vi "FPGA Time Management.vi"   [LabVIEW 2020]
uses:
  <vilib>/Platform/TimedLoop/XDataNode/timing_clust.ctl
  <vilib>/Platform/TimedLoop/XDataNode/nitl_modes.ctl
  <vilib>/Platform/TimedLoop/XDataNode/wakeup.ctl
  <vilib>/rvi/Emulation/niFpgaGetClockAttributes.vi
  <vilib>/rvi/Emulation/niFpgaSctlEmulationGetInTimedLoop.vi
  <vilib>/rvi/Emulation/niFpgaEmulationReportErrorSimple.vi
  <vilib>/rvi/eio/common/nirviEmuTemplateMethod_errors.vi
  <vilib>/rvi/eio/common/nirviEmuTemplatePropertyGet_noerrors.vi
  Front Panel Globals.vi
  <vilib>/rvi/Emulation/niFpgaProcessEmulError.vi
  <vilib>/rvi/Emulation/niFpgaCriticalErrorInLSC.vi
  <vilib>/eio/EIOMethodNode/EIOMethodNode.xnode
  <vilib>/eio/EIOPropertyNode/EIOPropertyNode.xnode
  <vilib>/LabVIEW Targets/FPGA/cRIO/shared/nicrio_ModuleControls/nicrio_cRIO-9467_Latitude.ctl
  <vilib>/LabVIEW Targets/FPGA/cRIO/shared/nicrio_ModuleControls/nicrio_cRIO-9467_Longitude.ctl
  <vilib>/LabVIEW Targets/FPGA/cRIO/shared/nicrio_ModuleControls/nicrio_cRIO-9467_Altitude.ctl
  <vilib>/platform/TimedLoop/XDataNode/XDataNode.xnode
  FPGA Timekeeper 1.1b0/FPGA Timekeeper.lvlib
  <vilib>/rvi/eio/common/nirviEmuTemplatePropertyGet_errors.vi
  <vilib>/rvi/eio/common/nirviEmuTemplatePropertySet_errors.vi
  <vilib>/rvi/eio/common/nirviEmuTemplatePropertySet_noerrors.vi
  <vilib>/Platform/TimedLoop/XDataNode/XDNodeRunTimeDep.lvlib
types:
  T1 = typedef "XDNodeRunTimeDep.lvlib/timing_clust.ctl" = cluster{"Expected End [f-1]":u64, "Actual End [f-1]":u64, "Finished Late? [f-1]":bool, "Expected End [i-1]":u64, "Actual End [i-1]":u64, "Finished Late? [i-1]":bool, "Expected Start [i]":u64, "Actual Start [i]":u64, "Expected Start [f]":u64, "Actual Start [f]":u64, "Source Name":string, "Structure Name":string, "Period":i64, "Deadline":i64, "Offset":i64, "Start":i64, "Priority":i32, "Timeout":i32, "Mode":T2, "Wakeup Reason":T3, "Error":errorcluster, "Source Type":string, "Secondary Source Type":string, "Global End Time":u64, "Global Start Time":u64, "Frame Duration":u64, "Iteration Duration":u64, "Assigned CPU":i32, "I/O Scan Engine Mode":u32}
  T2 = typedef "XDNodeRunTimeDep.lvlib/nitl_modes.ctl" = enum32{"No Change", "Process missed periods, maintain original phase", "Discard missed periods, maintain original phase", "Process missed periods, ignore original phase", "Discard missed periods, ignore original phase"}
  T3 = typedef "XDNodeRunTimeDep.lvlib/wakeup.ctl" = enum32{"Normal", "Aborted", "Asynchronous wakeup", "Timing source error", "Timed loop error", "Timeout"}
  T4 = enum8{"Initializing", "Normal", "Unable to get fix"}
  T5 = enum8{"Unknown", "Normal", "Absent", "Overcurrent"}
  T6 = typedef "nicrio_cRIO-9467_Latitude.ctl" = fxp<+/-,28,8>
  T7 = typedef "nicrio_cRIO-9467_Longitude.ctl" = fxp<+/-,29,9>
  T8 = typedef "nicrio_cRIO-9467_Altitude.ctl" = fxp<+/-,24,17>
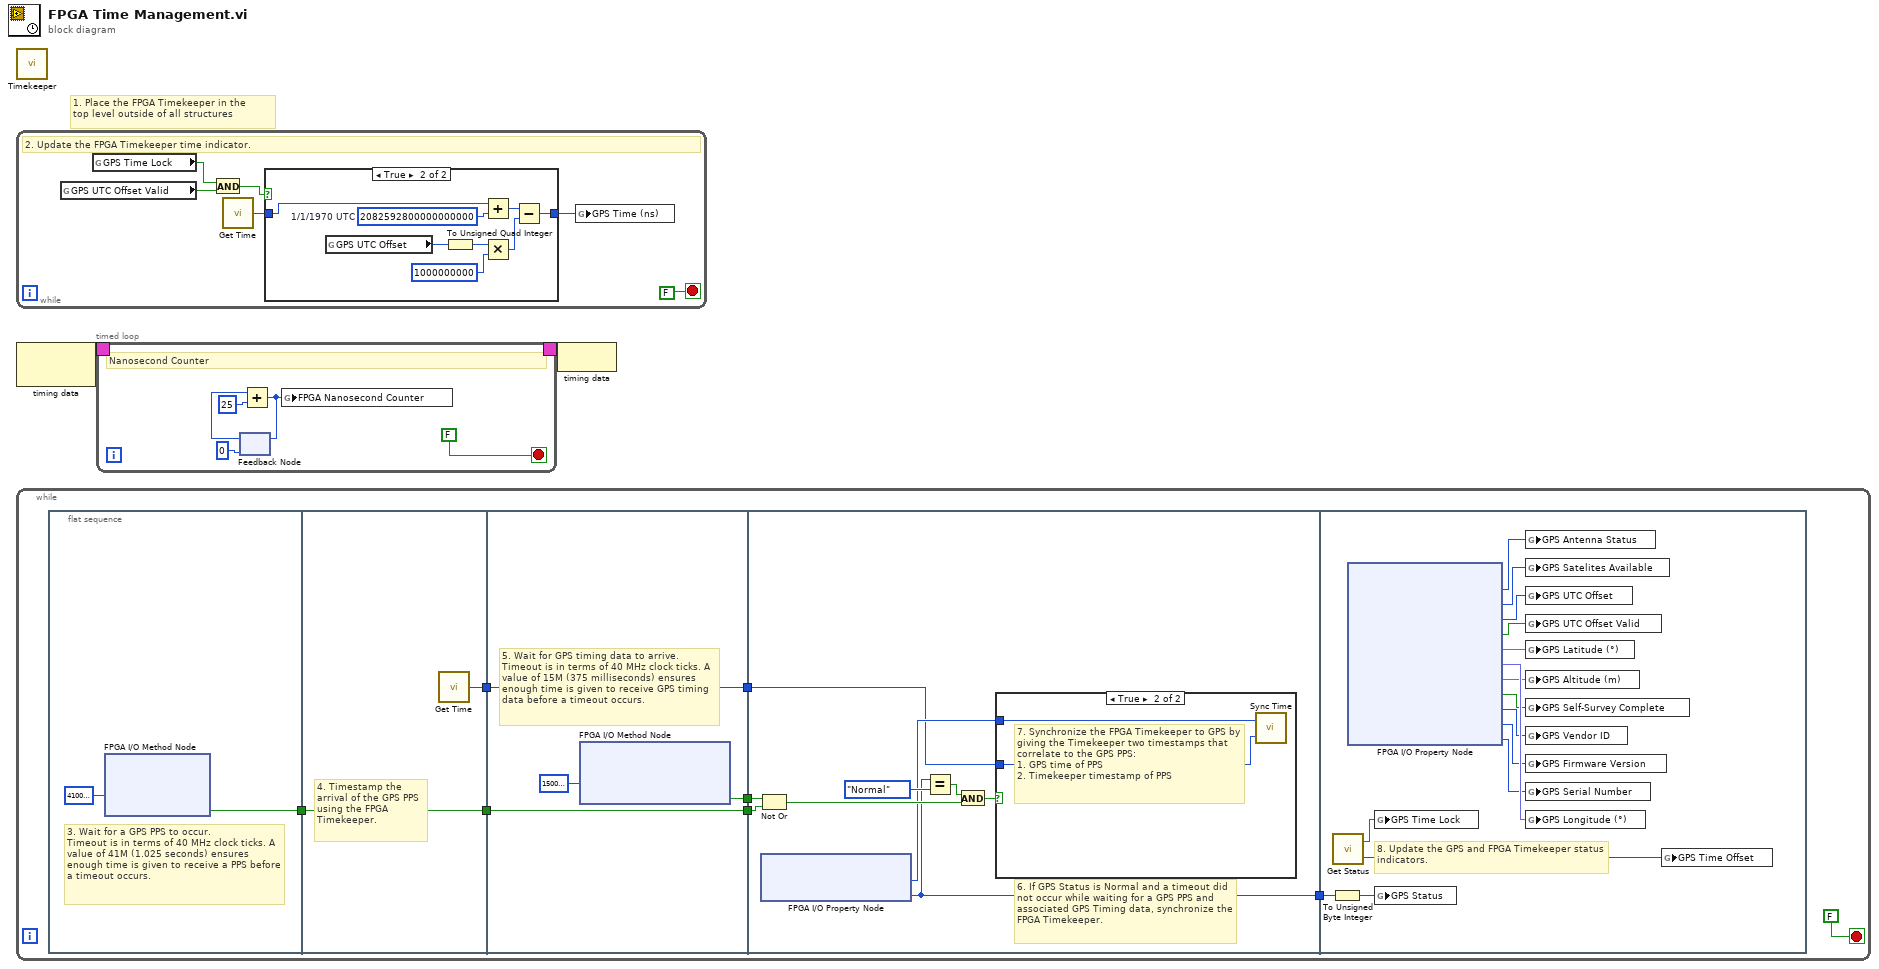
[diagram p0: block diagram]
diagram:
  # "1. Place the FPGA Timekeeper in the\ntop level outside of all structures"
  n1 = call "Timekeeper.vi"() -> ()  [unwired: 12 in]
  n2 = while {
    stop <- FALSE stop-if-true
    # "2. Update the FPGA Timekeeper time indicator."
    n3 = global read "Front Panel Globals.vi" "GPS UTC Offset Valid"() -> (w4:bool)
    n4 = global read "Front Panel Globals.vi" "GPS Time Lock"() -> (w5:bool)
    n5 = And(x=w5, y=w4) -> (x .and. y?=w3:bool)
    n6 = call "Get Time.vi"() -> ("time (ns)"=w7:u64)
    n7 = case shown="True" w3 {
      tunnel: w7 -> [w9 w17]
      tunnel: [w9 w11] -> w6
      frame False {
      }
      frame True {
        w10 = u64 2082592800000000000  # 1/1/1970 UTC
        n8 = global read "Front Panel Globals.vi" "GPS UTC Offset"() -> (w16:i8)
        n9 = To Unsigned Quad Integer(1:w16) -> (0:w15:u64)
        n10 = Add(x=w17, y=w10) -> (x+y=w13:u64)
        n11 = Multiply(x=w15, y=u64 1000000000) -> (x*y=w12:u64)
        n12 = Subtract(x=w13, y=w12) -> (x-y=w11:u64)
      }
    }
    n13 = global write "Front Panel Globals.vi" "GPS Time (ns)"(w6) -> ()
  }
  n14 = node-c288() -> (w2:T1)  [unwired: 1 in]
  n15 = while {
    stop <- FALSE stop-if-true
    n16 = flat-sequence {
      tunnel: [w26] -> w24
      tunnel: w24 -> [w29]
      tunnel: [w29] -> w23
      tunnel: [w28] -> w21
      tunnel: [w32] -> w25
      tunnel: w23 -> [w31]
      tunnel: [w31] -> w22
      tunnel: w21 -> [w30]
      tunnel: [w30] -> w20
      tunnel: w25 -> [w41]
      tunnel: w22 -> [w40]
      tunnel: w20 -> [w35]
      tunnel: [w34] -> w19
      tunnel: w19 -> [w59]
      frame #0 {
        # "3. Wait for a GPS PPS to occur.\nTimeout is in terms of 40 MHz clock ticks. A value of 41M (1.025 seconds) ensures enough time is given to receive a PPS before a timeout occurs."
        n17 = xnode "FPGA I/O Method Node"("Timeout"=41000000) -> ("Timed Out"=w26:bool)  [unwired: 1 in, 1 out]
      }
      frame #1 {
        # "4. Timestamp the arrival of the GPS PPS using the FPGA Timekeeper."
        n18 = call "Get Time.vi"() -> ("time (ns)"=w28:u64)
      }
      frame #2 {
        # "5. Wait for GPS timing data to arrive.\nTimeout is in terms of 40 MHz clock ticks. A value of 15M (375 milliseconds) ensures enough time is given to receive GPS timing data before a timeout occurs."
        n19 = xnode "FPGA I/O Method Node"("Timeout"=15000000) -> ("Timed Out"=w32:bool)  [unwired: 1 in, 1 out]
      }
      frame #3 {
        # "6. If GPS Status is Normal and a timeout did not occur while waiting for a GPS PPS and associated GPS Timing data, synchronize the FPGA Timekeeper."
        n20 = Not Or(1:w40, 2:w41) -> (0:w38:bool)
        n21 = xnode "FPGA I/O Property Node"() -> ("PPS Timestamp (TAI)"=w36:u64, "GPS Status"=w34:T4)  [unwired: 1 in, 1 out]
        n22 = Equal?(x=w34, y=T4."Normal") -> (x = y?=w39:bool)
        n23 = And(x=w39, y=w38) -> (x .and. y?=w37:bool)
        n24 = case shown="True" w37 {
          tunnel: w36 -> [_ w44]
          tunnel: w35 -> [_ w43]
          frame False {
          }
          frame True {
            # "7. Synchronize the FPGA Timekeeper to GPS by giving the Timekeeper two timestamps that correlate to the GPS PPS:\n1. GPS time of PPS\n2. Timekeeper timestamp of PPS"
            n25 = call "Sync Time.vi"("FPGA Timekeeper time (ns)"=w43, "time reference time (ns)"=w44) -> ()
          }
        }
      }
      frame #4 {
        # "8. Update the GPS and FPGA Timekeeper status indicators."
        n26 = To Unsigned Byte Integer(number=w59) -> (unsigned 8bit integer=w52:u8)
        n27 = call "Get Status.vi"() -> ("FPGA Timekeeper locked"=w57:bool, "offset from time reference"=w58:i32)
        n28 = xnode "FPGA I/O Property Node"() -> ("Antenna Status"=w53:T5, "Satellites Available"=w54:u8, "UTC Offset"=w55:i8, "UTC Offset Valid"=w56:bool, "Latitude (°)"=w51:T6, "Longitude (°)"=w50:T7, "Altitude (m)"=w49:T8, "Self-Survey Complete"=w46:bool, "Vendor ID"=w48:u16, "Firmware Version"=w47:u32, "Serial Number"=w45:u32)  [unwired: 1 in, 1 out]
        n29 = global write "Front Panel Globals.vi" "GPS Time Lock"(w57) -> ()
        n30 = global write "Front Panel Globals.vi" "GPS Status"(w52) -> ()
        n31 = global write "Front Panel Globals.vi" "GPS Antenna Status"(w53) -> ()
        n32 = global write "Front Panel Globals.vi" "GPS Satelites Available"(w54) -> ()
        n33 = global write "Front Panel Globals.vi" "GPS UTC Offset"(w55) -> ()
        n34 = global write "Front Panel Globals.vi" "GPS UTC Offset Valid"(w56) -> ()
        n35 = global write "Front Panel Globals.vi" "GPS Latitude (°)"(w51) -> ()
        n36 = global write "Front Panel Globals.vi" "GPS Altitude (m)"(w49) -> ()
        n37 = global write "Front Panel Globals.vi" "GPS Self-Survey Complete"(w46) -> ()
        n38 = global write "Front Panel Globals.vi" "GPS Vendor ID"(w48) -> ()
        n39 = global write "Front Panel Globals.vi" "GPS Firmware Version"(w47) -> ()
        n40 = global write "Front Panel Globals.vi" "GPS Serial Number"(w45) -> ()
        n41 = global write "Front Panel Globals.vi" "GPS Longitude (°)"(w50) -> ()
        n42 = global write "Front Panel Globals.vi" "GPS Time Offset"(w58) -> ()
      }
    }
  }
  n43 = timed-loop {
    timing: w2 -> [_]
    timing-out: [_] -> w1
    stop <- FALSE stop-if-true
    # "Nanosecond Counter"
    n44 = feedback #1(i64 0) -> (w63:i64)
    n45 = Add(x=w63, y=i64 25) -> (x+y=w60:i64)
    n46 = feedback-in #1(w60) -> ()
    n47 = global write "Front Panel Globals.vi" "FPGA Nanosecond Counter"(w60) -> ()
  }
  n48 = node-c288(w1) -> ()
